vi "Test 2.vi"() -> ()   [LabVIEW 2015, in "Drona basic.lvlib"]
uses:
  Drona basic.lvlib
panel:
  in  "Boolean":bool
  in  "Listbox":i32(listbox)
  in  "Ring":u16(ring)
  in  "Numeric 4":dbl
  in  "Numeric 3":dbl
  in  "Numeric 2":dbl
  in  "Numeric":dbl
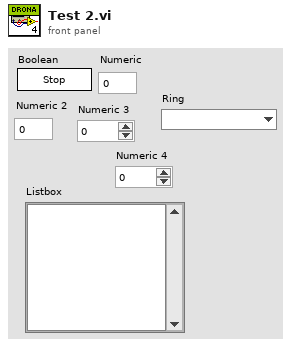
[diagram p1: front panel]
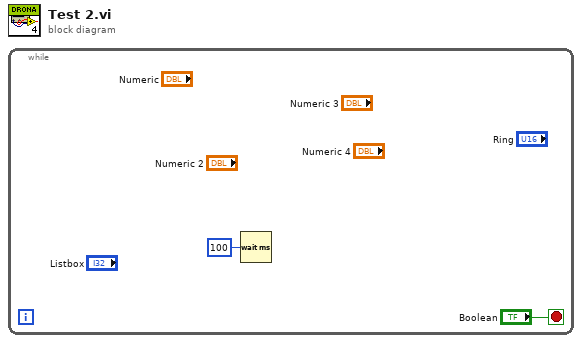
[diagram p0: block diagram]
diagram:
  n1 = while {
    stop <- "Boolean" stop-if-true
    n2 = Wait (ms)(milliseconds to wait=u32 100) -> ()  [unwired: 1 out]
  }
